vi "Format String Get Modifiers.vi"(11 "Start String":string) -> (0 "Min Width":u16, 1 "Precision":i32, 2 "Code Character":string, 3 "Modifiers":string, 4 "Error":bool, 5 "Remaining String":string)   [LabVIEW 2018, in "Numeric Data Type.lvclass"]
uses:
  Numeric Data Type.lvclass
panel:
  out "*(type *) &x":u8[](array[numeric])
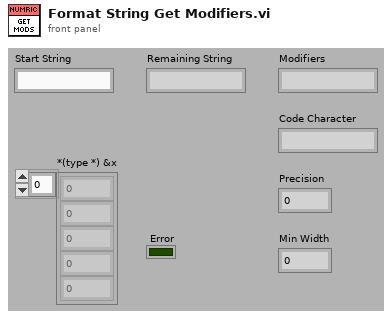
[diagram p1: front panel]
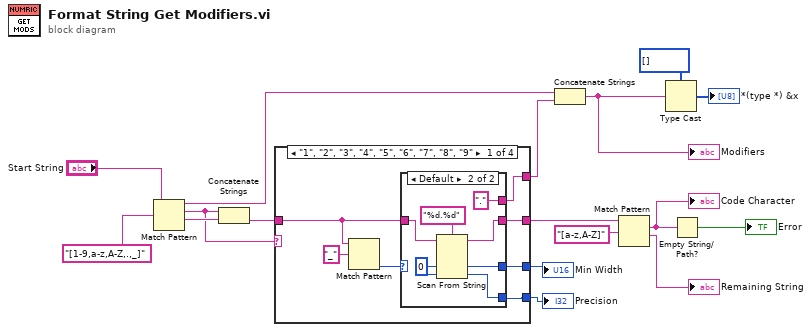
[diagram p0: block diagram]
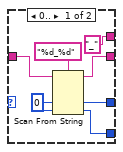
[diagram p2: hidden frame]
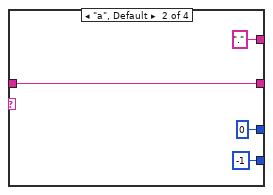
[diagram p3: hidden frame]
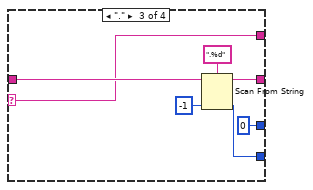
[diagram p4: hidden frame]
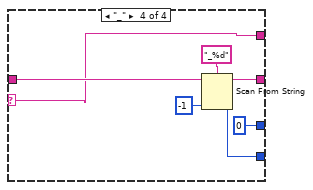
[diagram p5: hidden frame]
diagram:
  n1 = Match Pattern(string="Start String", regular expression="[1-9,a-z,A-Z,.,_]") -> (before substring=w5:string, match substring=w11:string, after substring=w15:string)  [unwired: 1 in, 1 out]
  n2 = Concatenate Strings(w11, w15) -> (w14:string)
  n3 = case shown="\"1\", \"2\", \"3\", \"4\", \"5\", \"6\", \"7\", \"8\", \"9\"" w11 {
    selector: w11 -> [_ _ w43 w50]
    tunnel: w14 -> [w21 w42 w49 w56]
    tunnel: [w24 -1 ("default value 1") w45 w52] -> w13
    tunnel: [w23 0 ("default value 1") 0 ("default value 1") 0 ("default value 1")] -> w12
    tunnel: [w22 w42 w47 w54] -> w9
    tunnel: [w18 "." w43 w50] -> w6
    frame "1", "2", "3", "4", "5", "6", "7", "8", "9" {
      n4 = Match Pattern(string=w21, regular expression="_") -> (offset past match=w19:i32)  [unwired: 1 in, 3 out]
      n5 = case shown="Default" w19 {
        tunnel: [w27 w36] -> w24
        tunnel: [w28 w35] -> w23
        tunnel: [w29 w34] -> w22
        tunnel: w21 -> [w26 w33]
        tunnel: ["_" "."] -> w18
        frame 0.. {
          w30 = 0 ("default value 1")
          n6 = Scan From String(format string="%d_%d", input string=w26, default 1=w30, default 2=w30) -> (remaining string=w29:string, output 1=w28:i32, output 2=w27:i32)  [unwired: 2 in, 2 out]
        }
        frame Default {
          w37 = 0 ("default value 1")
          n7 = Scan From String(format string="%d.%d", input string=w33, default 1=w37, default 2=w37) -> (remaining string=w34:string, output 1=w35:i32, output 2=w36:i32)  [unwired: 2 in, 2 out]
        }
      }
    }
    frame "a", Default {
    }
    frame "." {
      n8 = Scan From String(format string=".%d", input string=w49, default 1=-1 ("default value 1")) -> (remaining string=w47:string, output 1=w45:i32)  [unwired: 2 in, 2 out]
    }
    frame "_" {
      n9 = Scan From String(format string="_%d", input string=w56, default 1=-1 ("default value 1")) -> (remaining string=w54:string, output 1=w52:i32)  [unwired: 2 in, 2 out]
    }
  }
  "Min Width" <- w12
  "Precision" <- w13
  n10 = Concatenate Strings(w5, w6) -> (w4:string)
  "Modifiers" <- w4
  n11 = Match Pattern(string=w9, regular expression="[a-z,A-Z]") -> (match substring=w1:string, after substring=→"Remaining String":string)  [unwired: 1 in, 2 out]
  "Code Character" <- w1
  n12 = Type Cast(type=u8[] [], x=w4) -> (*(type *) &x=→"*(type *) &x":u8[])
  n13 = Empty String/Path?(string/path=w1) -> (empty?=→"Error":bool)
